vi "demo - FSM automated test.vi"() -> ()   [LabVIEW 2024]
doc: "#vi_description \nUses the FSM template to execute a large lab operation of taking prompting users, taking measurements, and storing data, demonstrating how to keep code onto one block diagram screen..\nThetic Engineering Ltd."
uses:
  <vilib>/Utility/sysdir.llb/System Directory Type.ctl
  <vilib>/Analysis/1siggen.llb/Ramp Pattern by Delta.vi
  <vilib>/Analysis/2dsp.llb/1D Cross Correlation (DBL).vi
  <vilib>/Analysis/NI_AALBase.lvlib
  <vilib>/Analysis/NI_AALPro.lvlib
panel:
  out "Progress":u8(slide) scale=0.0..10.0
  out "Oven warmup":dbl(graph)
  out "Time Stamp":timestamp format="%<%x %.3X>T"
  out "User":string
  out "Data File":path
  out "Instrument 1":dbl(graph)
  out "Instrument 2":dbl(graph)
  out "Final":dbl[](graph)
  out "Correlation":dbl[](graph)
  # "Preparation"
  # "Data Capture"
  # "Data Analysis"
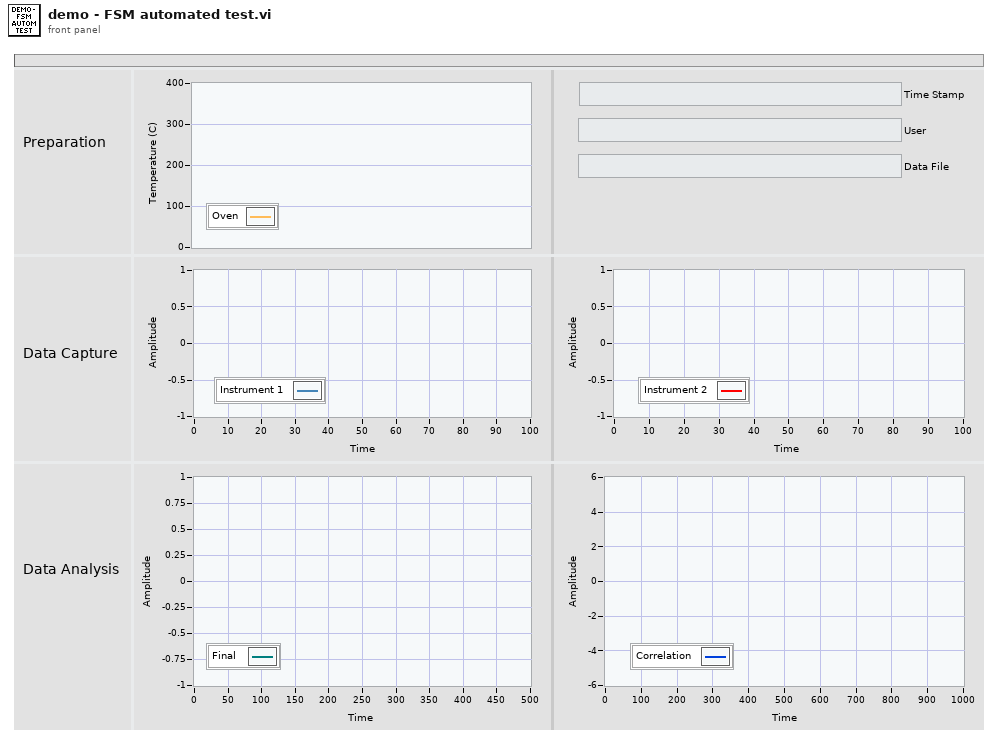
[diagram p1: front panel]
types:
  T1 = cluster{"datapoints":i32, "user":string, "boolean":bool, "file refnum":refnum<file>, "oven C":i32, "variant":string, "results 1":dbl[], "results 2":dbl[], "final data":dbl[]}
  T2 = enum16{"open", "replace", "create", "open or create", "replace or create", "replace or create with confirmation"}
  T3 = typedef "System Directory Type.ctl" = i32
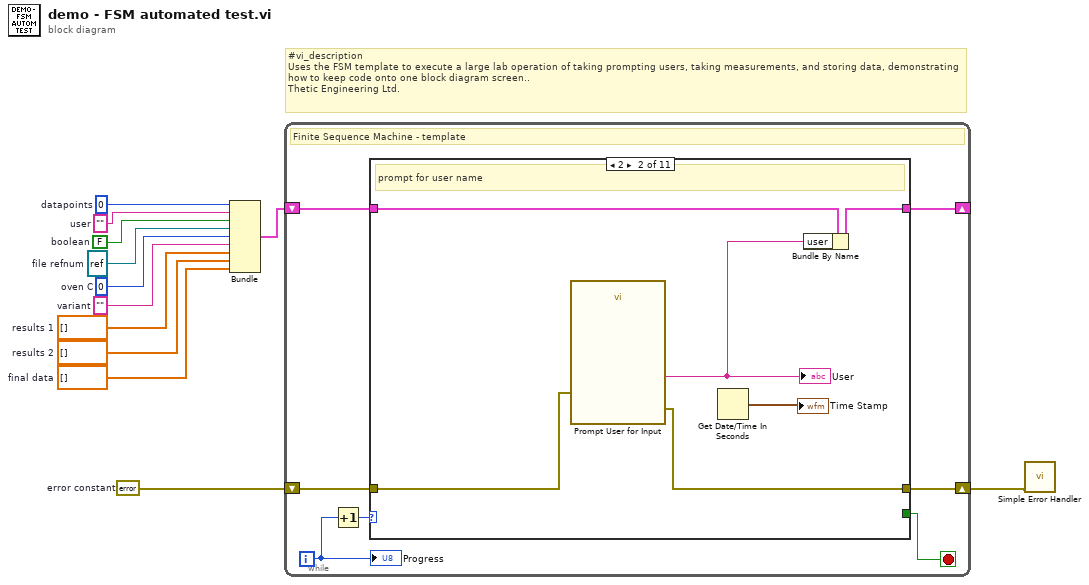
[diagram p0: block diagram]
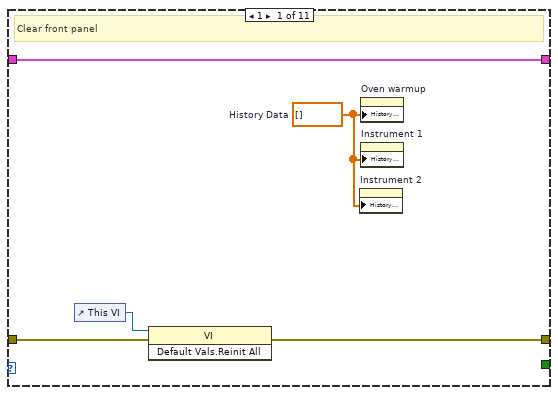
[diagram p2: hidden frame]
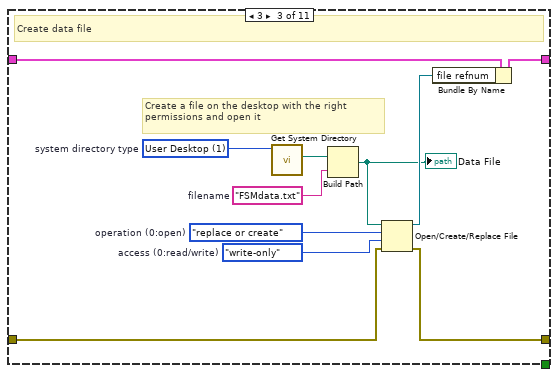
[diagram p3: hidden frame]
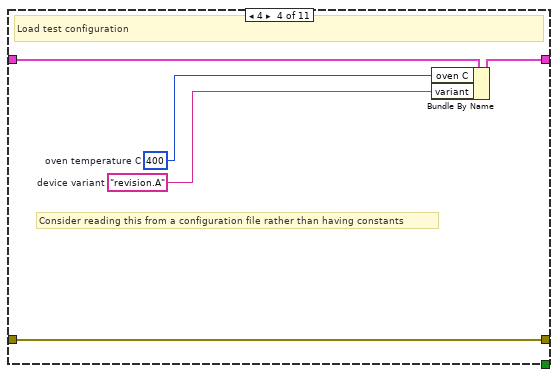
[diagram p4: hidden frame]
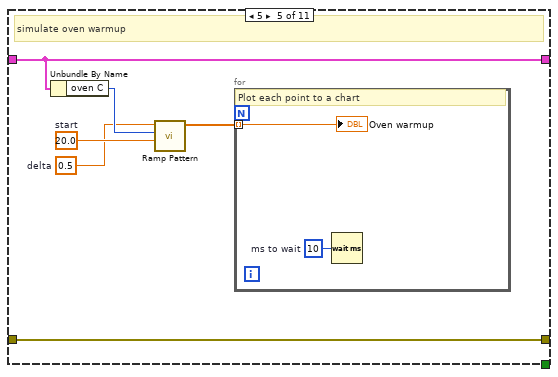
[diagram p5: hidden frame]
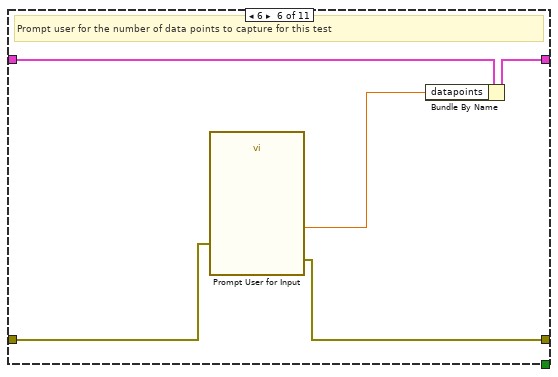
[diagram p6: hidden frame]
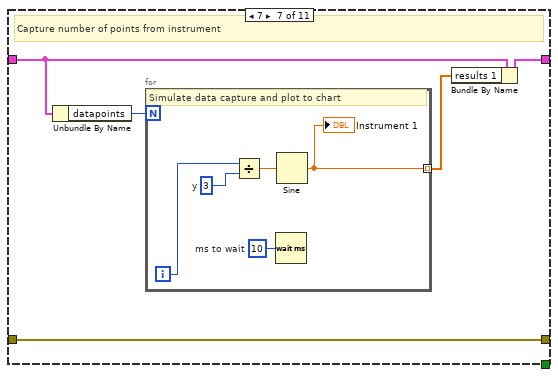
[diagram p7: hidden frame]
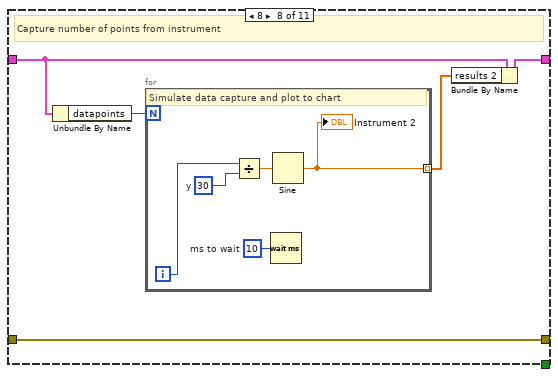
[diagram p8: hidden frame]
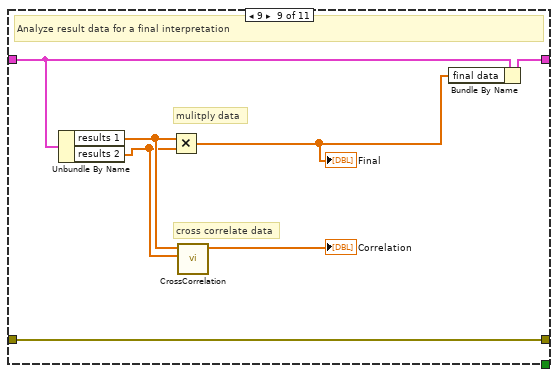
[diagram p9: hidden frame]
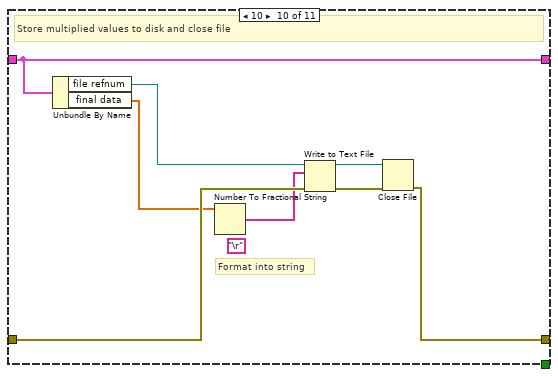
[diagram p10: hidden frame]
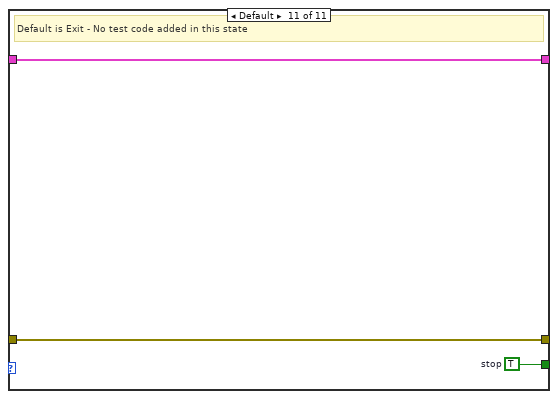
[diagram p11: hidden frame]
diagram:
  w2 = dbl[] []  # final data
  w3 = dbl[] []  # results 2
  w4 = dbl[] []  # results 1
  w5 = ""  # variant
  w6 = 0  # oven C
  w7 = refnum<file> refnum  # file refnum
  w8 = FALSE  # boolean
  w9 = ""  # user
  w10 = 0  # datapoints
  w12 = errorcluster {"status"=FALSE, "code"=0, "source"=""}  # error constant
  # "#vi_description \nUses the FSM template to execute a large lab operation of taking prompting users, taking measurements, and storing data, demonstrating how to keep code onto one block diagram screen..\nThetic Engineering Ltd."
  n1 = Bundle("datapoints"=w10, "user"=w9, "boolean"=w8, "file refnum"=w7, "oven C"=w6, "variant"=w5, "results 1"=w4, "results 2"=w3, "final data"=w2) -> (w11:T1)  [unwired: 1 in]
  n2 = while {
    shift-right: [w17] -> w1
    shift-left: w12 -> [w18]
    shift-right: [w16] -> _
    shift-left: w11 -> [w15]
    i -> [w13]
    stop <- w19 stop-if-true
    # "Finite Sequence Machine - template"
    n3 = Increment(x=w13) -> (x+1=w14:i32)
    n4 = case shown="2" w14 {
      tunnel: [_ _ _ _ _ _ _ _ _ _ w97] -> w19
      tunnel: w18 -> [w24 w28 w33 w46 w52 w56 w64 w74 w86 w93 w96]
      tunnel: [w21 w27 w32 w46 w52 w55 w64 w74 w86 w88 w96] -> w17
      tunnel: [w23 w29 w41 w44 w51 w58 w61 w71 w84 w94 w95] -> w16
      tunnel: w15 -> [w23 w30 w40 w45 w51 w59 w63 w73 w85 w94 w95]
      frame 1 {
        w22 = dbl[] []  # History Data
        # "Clear front panel"
        n5 = control-ref of="This VI"() -> (w20:refnum<vi>)
        n6 = invoke class="VI" method="Default Vals.Reinit All"(reference=w20, error in=w24) -> (error out=w21:errorcluster)  [unwired: 1 in, 2 out]
        n7 = property on="Instrument 2" class="WFChart (strict)"("History Data"=w22) -> ()  [unwired: 2 in, 2 out]
        n8 = property on="Oven warmup" class="WFChart (strict)"("History Data"=w22) -> ()  [unwired: 2 in, 2 out]
        n9 = property on="Instrument 1" class="WFChart (strict)"("History Data"=w22) -> ()  [unwired: 2 in, 2 out]
      }
      frame 2 {
        # "prompt for user name"
        n10 = call "Prompt User for Input"("error in (no error)"=w28) -> ("user"=w26:string, "error out"=w27:errorcluster)  [unwired: 16 in, 1 out]
        "User" <- w26
        n11 = Get Date/Time In Seconds() -> (seconds since 1Jan1904=→"Time Stamp":timestamp)
        n12 = Bundle By Name(cluster=w30, "user"=w26) -> (w29:T1)
      }
      frame 3 {
        w35 = "FSMdata.txt"  # filename
        w36 = enum16{"read/write", "read-only", "write-only"}."write-only"  # access (0:read/write)
        w37 = T2."replace or create"  # operation (0:open)
        w39 = T3 1 items=["User Home"=0, "User Desktop"=1, "User Documents"=2, "User Application Data"=3, "User Preferences"=4, "User Temporary"=5, "Public Documents"=6, "Public Application Data"=7, "Public Preferences"=8, "Public Cache"=13, "System Core Libraries"=9, "System Installed Libraries"=10, "Application Files"=11, "Boot Volume Root"=12]  # system directory type
        # "Create a file on the desktop with the right permissions and open it"
        # "Create data file"
        n13 = call <vilib>:"Get System Directory.vi"("system directory type"=w39) -> ("system directory"=w38:path)  [unwired: 10 in]
        n14 = Build Path(base path=w38, name or relative path=w35) -> (appended path=w31:path)
        "Data File" <- w31
        n15 = Open/Create/Replace File(file path (use dialog)=w31, error in=w33, operation (0:open)=w37, access (0:read/write)=w36) -> (refnum out=w34:refnum<file>, error out=w32:errorcluster)  [unwired: 2 in, 1 out]
        n16 = Bundle By Name(cluster=w40, "file refnum"=w34) -> (w41:T1)
      }
      frame 4 {
        w42 = "revision.A"  # device variant
        w43 = 400  # oven temperature C
        # "Consider reading this from a configuration file rather than having constants"
        # "Load test configuration"
        n17 = Bundle By Name(cluster=w45, "oven C"=w43, "variant"=w42) -> (w44:T1)
      }
      frame 5 {
        w48 = 0.5  # delta
        w49 = 20.0  # start
        # "simulate oven warmup"
        n18 = Unbundle By Name(w51) -> ("oven C"=w50:i32)
        n19 = call-poly <vilib>:"Ramp Pattern.vi"("start"=w49, "end"=w50, "delta"=w48) -> ("Ramp Pattern"=w47:dbl[])  [unwired: 6 in, 2 out]
        n20 = for {
          tunnel: w47 -> [w53] mode=indexing
          w54 = u32 10  # ms to wait
          # "Plot each point to a chart"
          n21 = Wait (ms)(milliseconds to wait=w54) -> ()  [unwired: 1 out]
          "Oven warmup" <- w53
        }
      }
      frame 6 {
        # "Prompt user for the number of data points to capture for this test"
        n22 = call "Prompt User for Input"("error in (no error)"=w56) -> ("datapoints"=w57:dbl, "error out"=w55:errorcluster)  [unwired: 16 in, 1 out]
        n23 = Bundle By Name(cluster=w59, "datapoints"=w57) -> (w58:T1)
      }
      frame 7 {
        # "Capture number of points from instrument"
        n24 = Unbundle By Name(w63) -> ("datapoints"=w62:i32)
        n25 = for {
          N: w62 -> [_]
          tunnel: [w65] -> w60 mode=indexing
          i -> [w67]
          w68 = 3  # y
          w69 = u32 10  # ms to wait
          # "Simulate data capture and plot to chart"
          n26 = Divide(x=w67, y=w68) -> (x/y=w66:dbl)
          n27 = Wait (ms)(milliseconds to wait=w69) -> ()  [unwired: 1 out]
          n28 = Sine(x=w66) -> (sin(x)=w65:dbl)
          "Instrument 1" <- w65
        }
        n29 = Bundle By Name(cluster=w63, "results 1"=w60) -> (w61:T1)
      }
      frame 8 {
        # "Capture number of points from instrument"
        n30 = Unbundle By Name(w73) -> ("datapoints"=w72:i32)
        n31 = for {
          N: w72 -> [_]
          tunnel: [w75] -> w70 mode=indexing
          i -> [w77]
          w78 = 30  # y
          w79 = u32 10  # ms to wait
          # "Simulate data capture and plot to chart"
          n32 = Divide(x=w77, y=w78) -> (x/y=w76:dbl)
          n33 = Wait (ms)(milliseconds to wait=w79) -> ()  [unwired: 1 out]
          n34 = Sine(x=w76) -> (sin(x)=w75:dbl)
          "Instrument 2" <- w75
        }
        n35 = Bundle By Name(cluster=w73, "results 2"=w70) -> (w71:T1)
      }
      frame 9 {
        # "cross correlate data"
        # "mulitply data"
        # "Analyze result data for a final interpretation"
        n36 = Unbundle By Name(w85) -> ("results 1"=w83:dbl[], "results 2"=w82:dbl[])
        n37 = Multiply(x=w83, y=w82) -> (x*y=w81:dbl[])
        "Final" <- w81
        n38 = call-poly <vilib>:"CrossCorrelation.vi"("Y"=w82, "X"=w83) -> ("Rxy"=→"Correlation":dbl[])  [unwired: 8 in, 1 out]
        n39 = Bundle By Name(cluster=w85, "final data"=w81) -> (w84:T1)
      }
      frame 10 {
        (unwired) "\r"
        # "Format into string"
        # "Store multiplied values to disk and close file"
        n40 = Unbundle By Name(w94) -> ("file refnum"=w92:refnum<file>, "final data"=w91:dbl[])
        n41 = Number To Fractional String(number=w91) -> (F-format string=w87:string[])  [unwired: 3 in]
        n42 = Write to Text File(file (use dialog)=w92, text=w87, error in=w93) -> (refnum out=w90:refnum<file>, error out=w89:errorcluster)  [unwired: 1 in, 1 out]
        n43 = Close File(refnum=w90, error in=w89) -> (error out=w88:errorcluster)  [unwired: 1 out]
      }
      frame Default {
        w97 = TRUE  # stop
        # "Default is Exit - No test code added in this state"
      }
    }
    "Progress" <- w13
  }
  n44 = call <vilib>:"Simple Error Handler.vi"("error in (no error)"=w1) -> ()  [unwired: 4 in, 5 out]
